vi "UMLEditor_LicenseAbout.vi"(0 "Header":string, 1 "Text":string="Copyright 2005 Endevo AB\nAll Rights Reserved\nProgrammed by\nMikael Holmström", 2 "FolderPath":path, 5 "error in (no error)":errorcluster) -> (19 "error out":errorcluster)   [LabVIEW 2016]
doc: "Helpinstructions."
panel:
  in  "Ok":bool
  out "Picture":picture
  out "Header info":string
  out "Program info":string
  out "UserInfo":string="UNREGISTERED"
  out "Key info":string
  out "ScrollText":string="Endevo is a modern swedish consulting company specialized in measurement systems involving high technical and social skills. We have officies in Stockholm, Gothenburg and Malmö. Visit us at: www.endevo.se"
  # "www.endevo.se\nsupport@endevo.se"
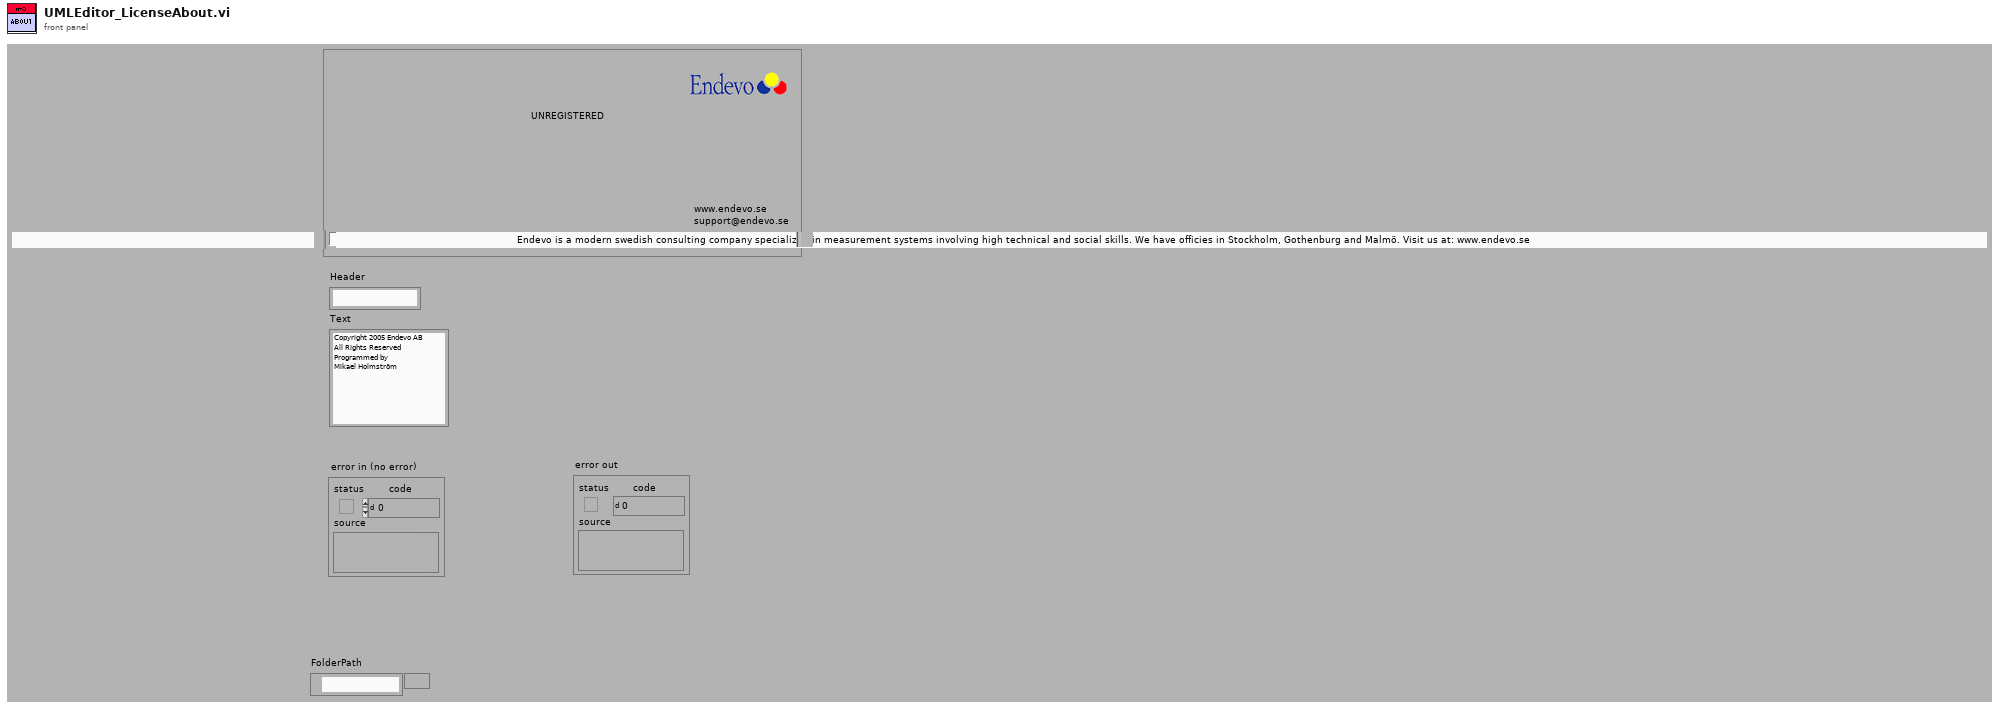
[diagram p1: front panel]
types:
  T1 = typedef "imagedata.ctl" = cluster{"image type":i32, "image depth":i32, "image":u8[], "mask":u8[], "colors":u32[], "Rectangle":cluster{"left":i16, "top":i16, "right":i16, "bottom":i16}}
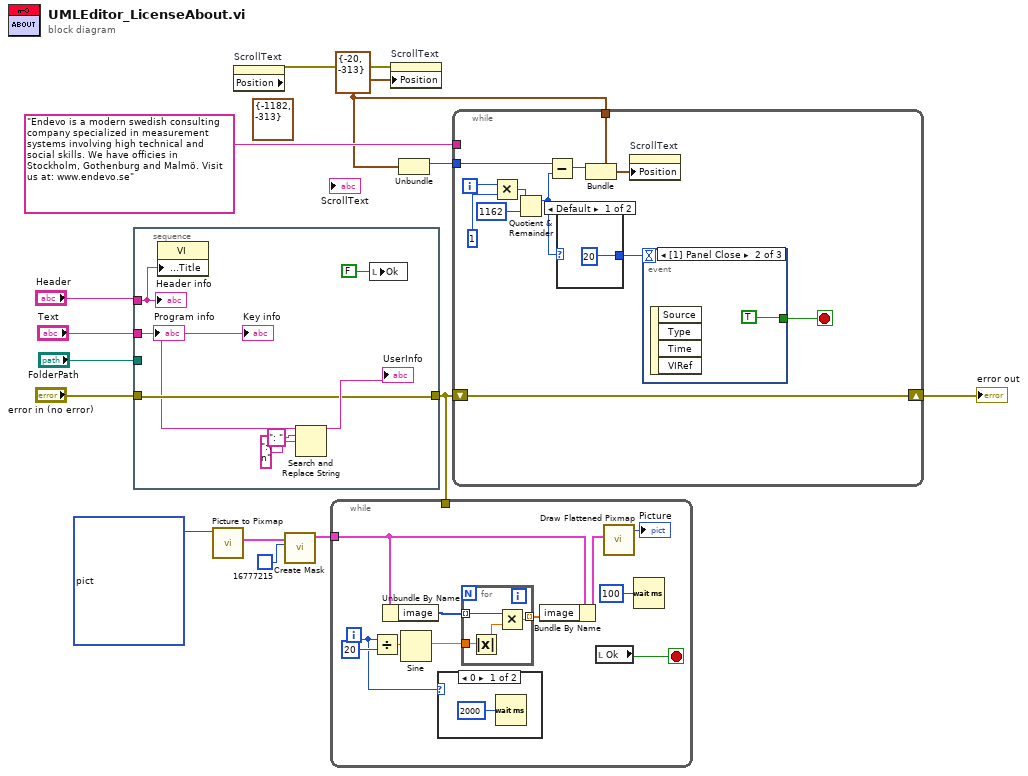
[diagram p0: block diagram]
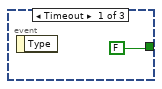
[diagram p3: hidden frame]
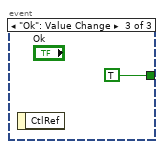
[diagram p4: hidden frame]
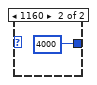
[diagram p5: hidden frame]
diagram:
  (unwired) cluster{"Left":i32, "Top":i32} {"Left"=-1182, "Top"=-313} ("Position")
  w7 = cluster{"Left":i32, "Top":i32} {"Left"=-20, "Top"=-313} ("Position")
  n1 = stacked-sequence {
    tunnel: [w16] -> w1
    tunnel: "error in (no error)" -> [w16]
    tunnel: "Text" -> [w15]
    tunnel: "Header" -> [w21]
    tunnel: "FolderPath" -> [_]
    frame #0 {
      n2 = property class="VI"("Front Panel Window:Title"=w21) -> ()  [unwired: 2 in, 2 out]
      n3 = Search and Replace String(input string=w15, search string=": ", replace string=":\n" ("replace string (\"\")")) -> (result string=→"UserInfo":string)  [unwired: 1 in, 7 out]
      n4 = local write "Ok"(FALSE ("Ok")) -> ()
      "Key info" <- w15
      "Program info" <- w15
      "Header info" <- w21
    }
  }
  n5 = call <vilib>:"Picture to Pixmap.vi"("picture"=picture bytes[29010] ("Picture")) -> ("image data"=w5:T1)  [unwired: 3 in, 7 out]
  n6 = property on="ScrollText" class="Str" props=["Position"]() -> (error out=w6:errorcluster)  [unwired: 2 in, 2 out]
  n7 = call <vilib>:"Create Mask.vi"("Mask Color (Black)"=u32 16777215, "image data"=w5) -> ("image data"=w2:T1)  [unwired: 2 in, 7 out]
  n8 = while {
    tunnel: w2 -> [w28]
    tunnel: w1 -> [_]
    i -> [w22]
    stop <- w23 stop-if-true
    n9 = Divide(x=w22, y=20) -> (x/y=w30:dbl)
    n10 = Unbundle By Name(w28) -> ("image"=w32:u8[])
    n11 = Sine(x=w30) -> (sin(x)=w26:dbl)
    n12 = case shown="0" w22 {
      frame 0 {
        n13 = Wait (ms)(milliseconds to wait=u32 2000) -> ()  [unwired: 1 out]
      }
      frame 1, Default {
      }
    }
    n14 = for {
      tunnel: w32 -> [w37] mode=indexing
      tunnel: [w36] -> w29 mode=indexing
      tunnel: w26 -> [w35]
      n15 = Absolute Value(x=w35) -> (abs(x)=w34:dbl)
      n16 = Multiply(x=w37, y=w34) -> (x*y=w36:dbl)
    }
    n17 = Bundle By Name(cluster=w28, "image"=w29) -> (w27:T1)
    n18 = local read "Ok"() -> (w23:bool)
    n19 = call <vilib>:"Draw Flattened Pixmap.vi"("image data"=w27) -> ("new picture"=→"Picture":picture)  [unwired: 1 in, 7 out]
    n20 = Wait (ms)(milliseconds to wait=u32 100) -> ()  [unwired: 1 out]
  }
  n21 = property on="ScrollText" class="Str"(error in=w6, "Position"=w7) -> ()  [unwired: 1 in, 2 out]
  n22 = Unbundle(w7) -> ("Left"=w8:i32)  [unwired: 1 out]
  n23 = while {
    tunnel: "Endevo is a modern swedish consulting company specialized in measurement systems involving high technical and social skills. We have officies in Stockholm, Gothenburg and Malmö. Visit us at: www.endevo.se" -> [_]
    shift-left: w1 -> [w49]
    shift-right: [w49] -> w14
    tunnel: w8 -> [w48]
    tunnel: w7 -> [w47]
    i -> [w43]
    stop <- w38 stop-if-true
    n24 = Multiply(x=w43, y=1 ("milliseconds to wait")) -> (x*y=w42:i32)
    n25 = Quotient & Remainder(x=w42, y=1162) -> (x-y*floor(x/y)=w40:i32)  [unwired: 1 out]
    n26 = Subtract(x=w48, y=w40) -> (x-y=w46:i32)
    n27 = case shown="Default" w40 {
      tunnel: [u32 20 ("milliseconds to wait") u32 4000 ("milliseconds to wait")] -> w39
      frame Default {
      }
      frame 1160 {
      }
    }
    n28 = Bundle(cluster=w47, "Left"=w46) -> (w45:cluster{"Left":i32, "Top":i32})  [unwired: 1 out]
    n29 = property on="ScrollText" class="Str"("Position"=w45) -> ()  [unwired: 2 in, 2 out]
    n30 = event shown="[1] Panel Close" {
      selector: _ -> [_ _ _]
      dyn-events: _ -> [_ _ _]
      timeout: w39 -> [_ _ _]
      tunnel: [FALSE ("Ok") TRUE ("Ok") TRUE ("Ok")] -> w38
      event Timeout {
        n31 = event-data() -> ()  [unwired: 2 out]
      }
      event Panel Close {
        n32 = event-data() -> ()  [unwired: 5 out]
      }
      event "Ok": Value Change {
        n33 = event-data() -> ()  [unwired: 2 out]
      }
    }
  }
  "error out" <- w14
